vi "send_data.vi"(1 "input 1":dbl) -> ()   [LabVIEW 2019]
uses:
  <vilib>/Platform/TimedLoop/XDataNode/timing_clust.ctl
  <vilib>/Platform/TimedLoop/XDataNode/nitl_modes.ctl
  <vilib>/Platform/TimedLoop/XDataNode/wakeup.ctl
  <vilib>/platform/TimedLoop/XDataNode/XDataNode.xnode
  <vilib>/Platform/TimedLoop/XDataNode/XDNodeRunTimeDep.lvlib
panel:
  out "input 2":dbl
  out "concatenated string":string
  out "error out":errorcluster
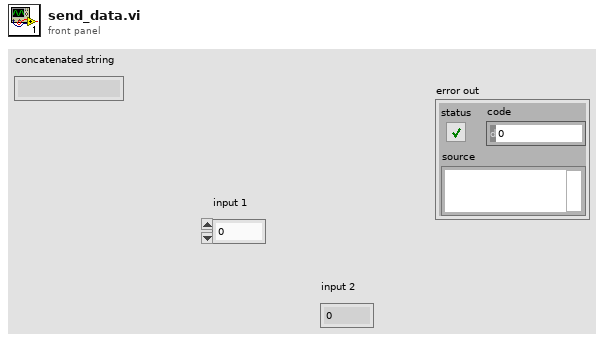
[diagram p1: front panel]
types:
  T1 = typedef "XDNodeRunTimeDep.lvlib/timing_clust.ctl" = cluster{"Expected End [f-1]":u64, "Actual End [f-1]":u64, "Finished Late? [f-1]":bool, "Expected End [i-1]":u64, "Actual End [i-1]":u64, "Finished Late? [i-1]":bool, "Expected Start [i]":u64, "Actual Start [i]":u64, "Expected Start [f]":u64, "Actual Start [f]":u64, "Source Name":string, "Structure Name":string, "Period":i64, "Deadline":i64, "Offset":i64, "Start":i64, "Priority":i32, "Timeout":i32, "Mode":T2, "Wakeup Reason":T3, "Error":errorcluster, "Source Type":string, "Secondary Source Type":string, "Global End Time":u64, "Global Start Time":u64, "Frame Duration":u64, "Iteration Duration":u64, "Assigned CPU":i32, "I/O Scan Engine Mode":u32}
  T2 = typedef "XDNodeRunTimeDep.lvlib/nitl_modes.ctl" = enum32{"No Change", "Process missed periods, maintain original phase", "Discard missed periods, maintain original phase", "Process missed periods, ignore original phase", "Discard missed periods, ignore original phase"}
  T3 = typedef "XDNodeRunTimeDep.lvlib/wakeup.ctl" = enum32{"Normal", "Aborted", "Asynchronous wakeup", "Timing source error", "Timed loop error", "Timeout"}
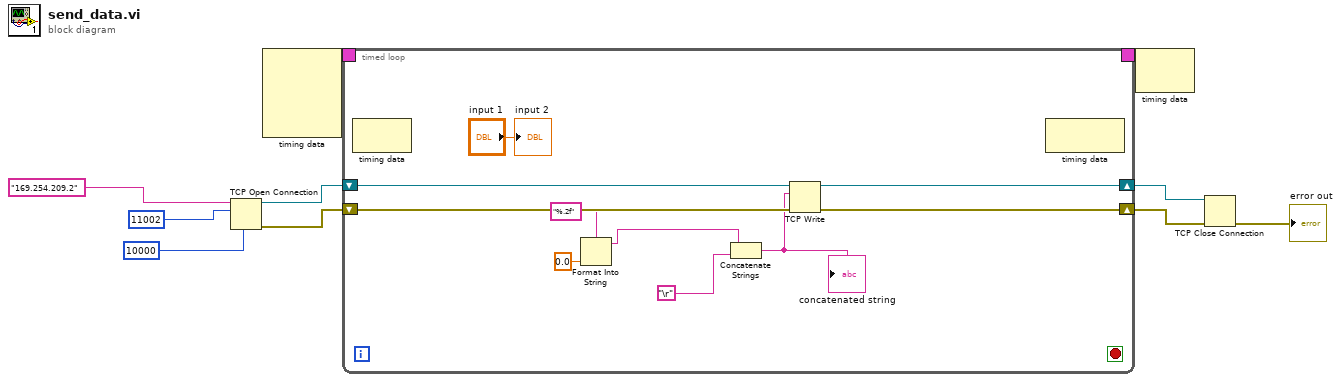
[diagram p0: block diagram]
diagram:
  n1 = TCP Open Connection(address="169.254.209.2" ("name"), remote port or service name=u16 11002, timeout ms (60000)=10000) -> (connection ID=w8:refnum<k5>, error out=w7:errorcluster)  [unwired: 2 in]
  n2 = node-c288() -> (w3:T1)  [unwired: 4 in]
  n3 = timed-loop {
    timing: w3 -> [_]
    timing-out: [_] -> w2
    shift-right: [w18] -> w6
    shift-left: w8 -> [w20]
    shift-right: [w17] -> w5
    shift-left: w7 -> [w19]
    stop <- _ stop-if-true
    n4 = node-c288() -> ()  [unwired: 1 in, 1 out]
    n5 = Format Into String(format string="%.2f", 0.0 ("input 1")) -> (resulting string=w14:string)  [unwired: 2 in, 1 out]
    n6 = Concatenate Strings(w14, "\r") -> (w15:string)
    "concatenated string" <- w15
    n7 = TCP Write(connection ID=w20, data in=w15, error in (no error)=w19) -> (connection ID out=w18:refnum<k5>, error out=w17:errorcluster)  [unwired: 1 in, 1 out]
    n8 = node-c288() -> ()  [unwired: 1 in, 1 out]
    "input 2" <- "input 1"
  }
  n9 = node-c288(w2) -> ()  [unwired: 1 out]
  n10 = TCP Close Connection(connection ID=w6, error in (no error)=w5) -> (error out=→"error out":errorcluster)  [unwired: 1 in, 1 out]
